vi "simple_RT_task.vi"(0 "stimulus length":u32=500 caption="Stimulus Length (ms)", 1 "monitor":u16 caption="Display", 5 "response window":u32=1000 caption="Response Window (ms)", 7 "ITI (ms)":u32=2000, 9 "file prefix":string caption="Output File Prefix", 11 "output folder":path caption="Output Folder", 12 "output channel":tag="Dev2/ao0" caption="Output Channel", 13 "randomization file":path) -> ()   [LabVIEW 2010]
uses:
  <vilib>/Utility/miscctls.llb/LVRectTypeDef.ctl
  <vilib>/Utility/miscctls.llb/LVPointTypeDef.ctl
  <vilib>/DAQmx/write.llb/DAQmx Write (Analog DBL 1Chan 1Samp).vi
  <vilib>/Utility/file.llb/Read From Spreadsheet File (DBL).vi
  <vilib>/DAQmx/create/channels.llb/DAQmx Create Channel (AO-Voltage-Basic).vi
  <vilib>/daqmx/miscellaneous.llb/DAQmx Fill In Error Info.vi
  <vilib>/Utility/inputDevices.llb/keyboardAcquire.vi
  <vilib>/Utility/inputDevices.llb/closeKeyboard.vi
panel:
  out "trial order":dbl[](array[numeric])
  out "old monitor":u16
  in  "Settings":enum32{"Page 1", "Page 2"}(tab)
  out "old panel bounds":T1
  out "output file ref":refnum<file>
  out "AO task id":refnum<k21>
  out "trial type":dbl
  out "response":T2(array[ring])
  out "response time":u32
  out "keyboard ID":refnum<k1>
  out "stimulus":string
  out "fixation":string
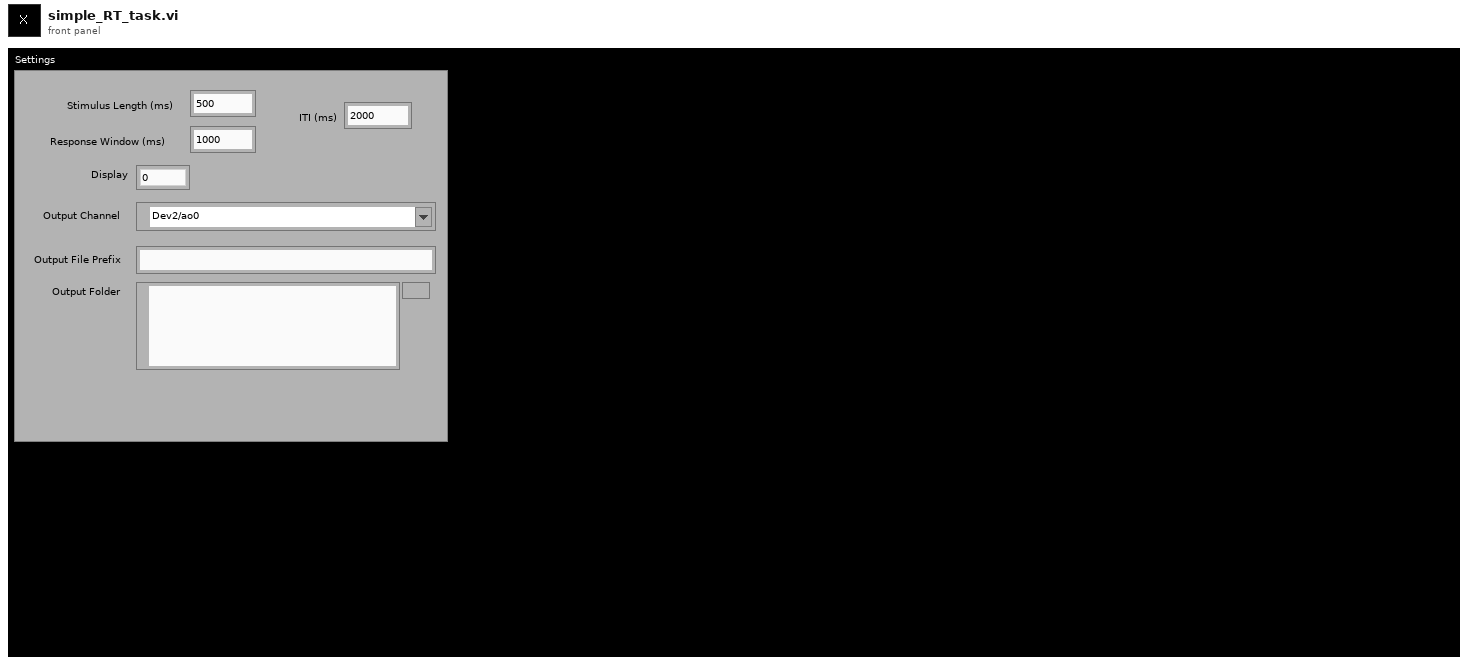
[diagram p1: front panel]
types:
  T1 = typedef "LVRectTypeDef.ctl" = cluster{"Left":i16, "Top":i16, "Right":i16, "Bottom":i16}
  T2 = enum16{"0", "1", "2", "3", "4", "5", "6", "7", "8", "9", "A", "B", "C", "D", "E", "F", "G", "H", "I", "J", "K", "L", "M", "N", "O", "P", "Q", "R", "S", "T", "U", "V", "W", "X", "Y", "Z", "F1", "F2", "F3", "F4", "F5", "F6", "F7", "F8", "F9", "F10", "F11", "F12", "F13", "F14", "F15", "ADD", "BACK", "BACKSLASH", "CAPITAL", "COMMA", "DECIMAL", "DELETE", "DIVIDE", "DOWN", "END", "EQUALS", "ESCAPE", "GRAVE (`)", "HOME", "INSERT", "LBRACKET", "LCONTROL", "LEFT", "L ALT", "LSHIFT", "LWIN", "MINUS", "MULTIPLY", "NEXT", "NUMLOCK", "NUMPAD_0", "NUMPAD_1", "NUMPAD_2", "NUMPAD_3", "NUMPAD_4", "NUMPAD_5", "NUMPAD_6", "NUMPAD_7", "NUMPAD_8", "NUMPAD_9", "PAUSE", "PERIOD", "PRIOR (PG UP)", "RBRACKET", "RCONTROL", "RETURN", "RIGHT", "R ALT", "RSHIFT", "RWIN", "SCROLL", "SEMICOLON", "SLASH", "SPACE", "SUBTRACT", "TAB", "UP", "ENTER (num pad)", "' (quote)"}[]
  T3 = enum16{"open", "replace", "create", "open or create", "replace or create", "replace or create with confirmation"}
  T4 = typedef "LVPointTypeDef.ctl" = cluster{"Horizontal":i16, "Vertical":i16}
  T5 = enum16{"0", "1", "2", "3", "4", "5", "6", "7", "8", "9", "A", "B", "C", "D", "E", "F", "G", "H", "I", "J", "K", "L", "M", "N", "O", "P", "Q", "R", "S", "T", "U", "V", "W", "X", "Y", "Z", "F1", "F2", "F3", "F4", "F5", "F6", "F7", "F8", "F9", "F10", "F11", "F12", "F13", "F14", "F15", "ADD", "BACK", "BACKSLASH", "CAPITAL", "COMMA", "DECIMAL", "DELETE", "DIVIDE", "DOWN", "END", "EQUALS", "ESCAPE", "GRAVE (`)", "HOME", "INSERT", "LBRACKET", "LCONTROL", "LEFT", "L ALT", "LSHIFT", "LWIN", "MINUS", "MULTIPLY", "NEXT", "NUMLOCK", "NUMPAD_0", "NUMPAD_1", "NUMPAD_2", "NUMPAD_3", "NUMPAD_4", "NUMPAD_5", "NUMPAD_6", "NUMPAD_7", "NUMPAD_8", "NUMPAD_9", "PAUSE", "PERIOD", "PRIOR (PG UP)", "RBRACKET", "RCONTROL", "RETURN", "RIGHT", "R ALT", "RSHIFT", "RWIN", "SCROLL", "SEMICOLON", "SLASH", "SPACE", "SUBTRACT", "TAB", "UP", "ENTER (num pad)", "' (quote)"}
  T6 = enum16{"big-endian, network order", "native, host order", "little-endian"}
  T7 = typedef "LVAllMonitorsDisplayTypeDef.ctl" = cluster{"Bounds":cluster{"Left":i16, "Top":i16, "Right":i16, "Bottom":i16}, "Depth":i16}[]
  T8 = cluster{"Bounds":cluster{"Left":i16, "Top":i16, "Right":i16, "Bottom":i16}, "Depth":i16}
  T9 = cluster{"Left":i16, "Top":i16, "Right":i16, "Bottom":i16}
  T10 = cluster{i32, "trial type":dbl, "response time":u32, "keyType 3":enum16{"0", "1", "2", "3", "4", "5", "6", "7", "8", "9", "A", "B", "C", "D", "E", "F", "G", "H", "I", "J", "K", "L", "M", "N", "O", "P", "Q", "R", "S", "T", "U", "V", "W", "X", "Y", "Z", "F1", "F2", "F3", "F4", "F5", "F6", "F7", "F8", "F9", "F10", "F11", "F12", "F13", "F14", "F15", "ADD", "BACK", "BACKSLASH", "CAPITAL", "COMMA", "DECIMAL", "DELETE", "DIVIDE", "DOWN", "END", "EQUALS", "ESCAPE", "GRAVE (`)", "HOME", "INSERT", "LBRACKET", "LCONTROL", "LEFT", "L ALT", "LSHIFT", "LWIN", "MINUS", "MULTIPLY", "NEXT", "NUMLOCK", "NUMPAD_0", "NUMPAD_1", "NUMPAD_2", "NUMPAD_3", "NUMPAD_4", "NUMPAD_5", "NUMPAD_6", "NUMPAD_7", "NUMPAD_8", "NUMPAD_9", "PAUSE", "PERIOD", "PRIOR (PG UP)", "RBRACKET", "RCONTROL", "RETURN", "RIGHT", "R ALT", "RSHIFT", "RWIN", "SCROLL", "SEMICOLON", "SLASH", "SPACE", "SUBTRACT", "TAB", "UP", "ENTER (num pad)", "' (quote)"}}
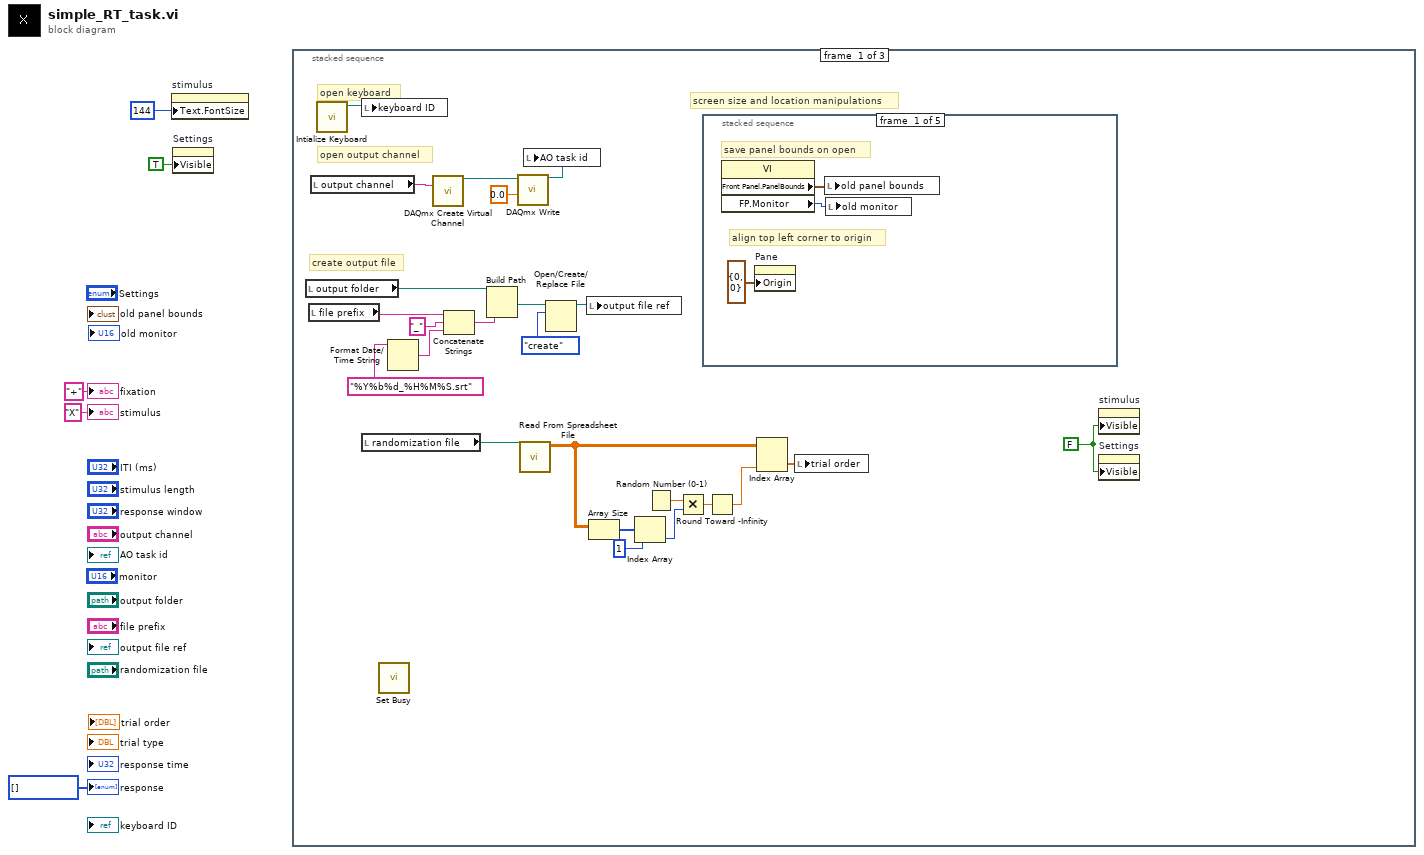
[diagram p0: block diagram]
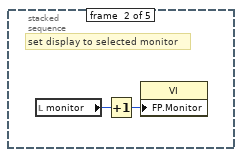
[diagram p2: hidden frame]
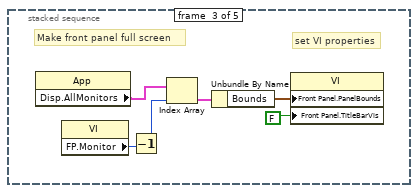
[diagram p3: hidden frame]
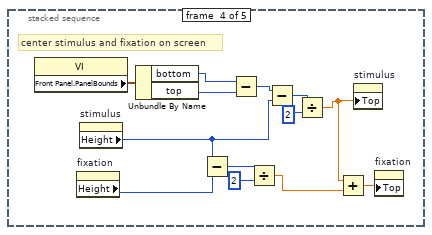
[diagram p4: hidden frame]
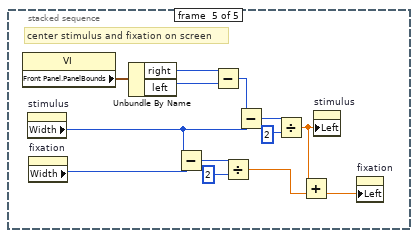
[diagram p5: hidden frame]
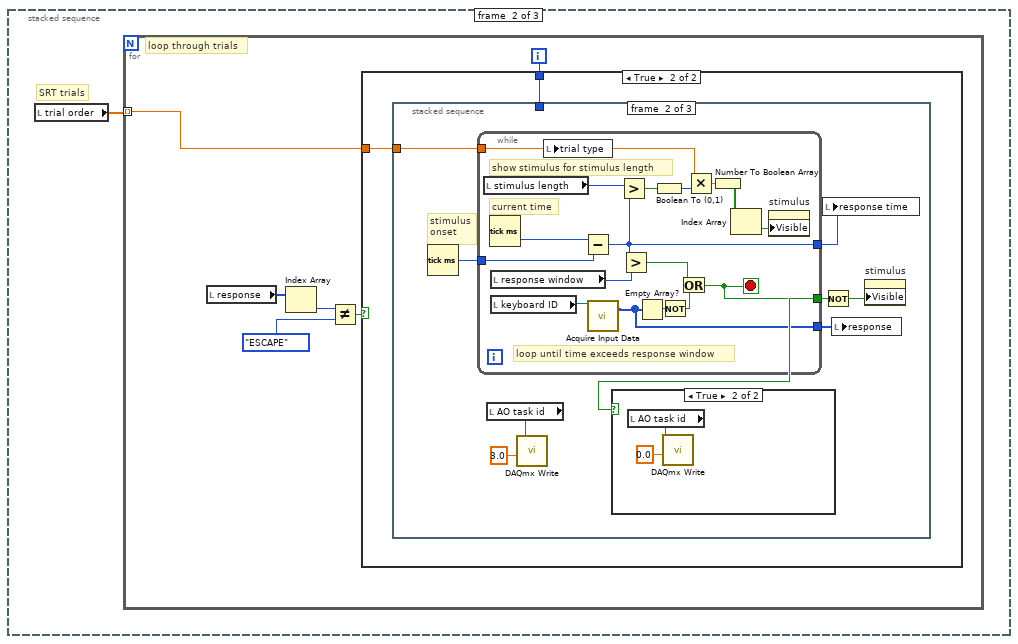
[diagram p6: hidden frame]
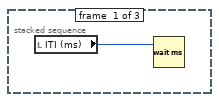
[diagram p8: hidden frame]
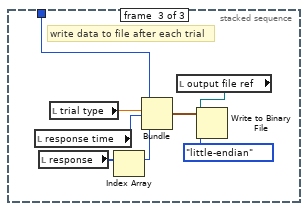
[diagram p10: hidden frame]
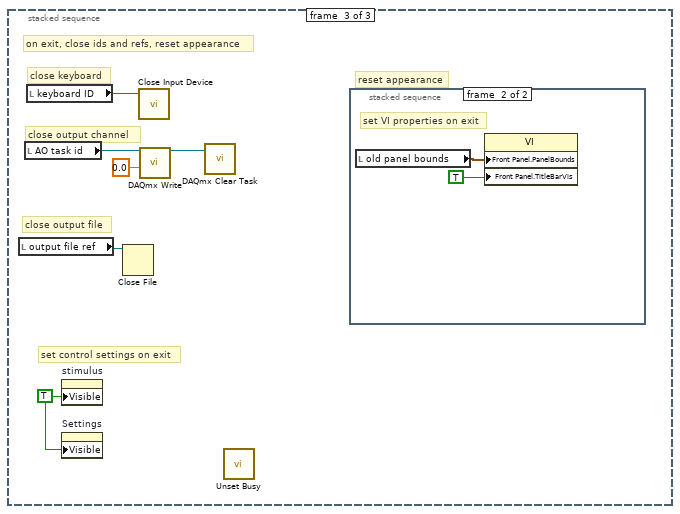
[diagram p11: hidden frame]
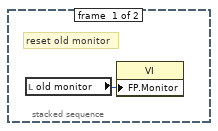
[diagram p12: hidden frame]
diagram:
  w1 = T2 [] items=["0", "1", "2", "3", "4", "5", "6", "7", "8", "9", "A", "B", "C", "D", "E", "F", "G", "H", "I", "J", "K", "L", "M", "N", "O", "P", "Q", "R", "S", "T", "U", "V", "W", "X", "Y", "Z", "F1", "F2", "F3", "F4", "F5", "F6", "F7", "F8", "F9", "F10", "F11", "F12", "F13", "F14", "F15", "ADD", "BACK", "BACKSLASH", "CAPITAL", "COMMA", "DECIMAL", "DELETE", "DIVIDE", "DOWN", "END", "EQUALS", "ESCAPE", "GRAVE (`)", "HOME", "INSERT", "LBRACKET", "LCONTROL", "LEFT", "L ALT", "LSHIFT", "LWIN", "MINUS", "MULTIPLY", "NEXT", "NUMLOCK", "NUMPAD_0", "NUMPAD_1", "NUMPAD_2", "NUMPAD_3", "NUMPAD_4", "NUMPAD_5", "NUMPAD_6", "NUMPAD_7", "NUMPAD_8", "NUMPAD_9", "PAUSE", "PERIOD", "PRIOR (PG UP)", "RBRACKET", "RCONTROL", "RETURN", "RIGHT", "R ALT", "RSHIFT", "RWIN", "SCROLL", "SEMICOLON", "SLASH", "SPACE", "SUBTRACT", "TAB", "UP", "ENTER (num pad)", "' (quote)"] ("response")
  n1 = property on="stimulus" class="Str"("Text.FontSize"=u32 144 ("Text.Font:Size")) -> ()  [unwired: 2 in, 2 out]
  n2 = property on="Settings" class="TabCtl (strict)"("Visible"=TRUE) -> ()  [unwired: 2 in, 2 out]
  n3 = stacked-sequence {
    frame #0 {
      w17 = FALSE ("Visible")
      # "screen size and location manipulations"
      # "create output file"
      # "open output channel"
      # "open keyboard"
      n4 = local read "output folder"() -> (w20:path)
      n5 = local read "file prefix"() -> (w21:string)
      n6 = local read "output channel"() -> (w27:tag)
      n7 = call <vilib>:"Intialize Keyboard.vi"() -> ("device ID"=w29:refnum<k1>)  [unwired: 10 in, 1 out]
      n8 = local write "keyboard ID"(w29) -> ()
      n9 = local read "randomization file"() -> (w12:path)
      n10 = call <vilib>:"Set Busy.vi"() -> ()  [unwired: 10 in, 2 out]
      n11 = Format Date/Time String(time format string (%c)="%Y%b%d_%H%M%S.srt") -> (date/time string=w7:string)  [unwired: 2 in]
      n12 = call-poly <vilib>:"DAQmx Create Virtual Channel.vi"("physical channels"=w27) -> ("task out"=w24:refnum<k21>)  [unwired: 13 in, 1 out]
      n13 = Concatenate Strings(w21, "_" ("string"), w7) -> (w19:string)
      n14 = Build Path(base path=w20, name or relative path=w19) -> (appended path=w18:path)
      n15 = call-poly <vilib>:"DAQmx Write.vi"("task/channels in"=w24, "data"=0.0) -> ("task out"=w23:refnum<k21>)  [unwired: 11 in, 2 out]
      n16 = call-poly <vilib>:"Read From Spreadsheet File.vi"("file path (dialog if empty)"=w12) -> ("all rows"=w11:dbl[][])  [unwired: 6 in, 4 out]
      n17 = local write "AO task id"(w23) -> ()
      n18 = Open/Create/Replace File(file path (use dialog)=w18, operation (0:open)=T3."create") -> (refnum out=w25:refnum<file>)  [unwired: 4 in, 2 out]
      n19 = local write "output file ref"(w25) -> ()
      n20 = Array Size(array=w11) -> (size(s)=w10:i32[])
      n21 = Index Array(array=w10, index=1) -> (element=w8:i32)
      n22 = Random Number (0-1)() -> (number: 0 to 1=w16:dbl)
      n23 = Multiply(x=w16, y=w8) -> (x*y=w15:dbl)
      n24 = stacked-sequence {
        frame #0 {
          # "align top left corner to origin"
          # "save panel bounds on open"
          n25 = property class="VI"() -> ("Front Panel.PanelBounds"=w32:T1, "FP.Monitor"=w30:u16)  [unwired: 2 in, 2 out]
          n26 = property on="Pane" class="Pane"("Origin"=T4 {"Horizontal"=0, "Vertical"=0}) -> ()  [unwired: 2 in, 2 out]
          n27 = local write "old panel bounds"(w32) -> ()
          n28 = local write "old monitor"(w30) -> ()
        }
        frame #1 {
          # "set display to selected monitor"
          n29 = local read "monitor"() -> (w34:u16)
          n30 = Increment(x=w34) -> (x+1=w33:u16)
          n31 = property class="VI"("FP.Monitor"=w33) -> ()  [unwired: 2 in, 2 out]
        }
        frame #2 {
          # "set VI properties"
          # "Make front panel full screen"
          n32 = property class="App"() -> ("Disp.AllMonitors"=w40:T7)  [unwired: 2 in, 2 out]
          n33 = property class="VI"() -> ("FP.Monitor"=w39:u16)  [unwired: 2 in, 2 out]
          n34 = Decrement(x=w39) -> (x-1=w38:u16)
          n35 = Index Array(array=w40, index=w38) -> (element=w37:T8)
          n36 = Unbundle By Name(w37) -> ("Bounds"=w36:T9)
          n37 = property class="VI"("Front Panel.PanelBounds"=w36, "Front Panel.TitleBarVis"=FALSE ("Front Panel Window:Title Bar Visible")) -> ()  [unwired: 2 in, 2 out]
        }
        frame #3 {
          # "center stimulus and fixation on screen"
          n38 = property class="VI"() -> ("Front Panel.PanelBounds"=w51:T1)  [unwired: 2 in, 2 out]
          n39 = property on="fixation" class="Str"() -> ("Height"=w44:u32)  [unwired: 2 in, 2 out]
          n40 = property on="stimulus" class="Str"() -> ("Height"=w45:u32)  [unwired: 2 in, 2 out]
          n41 = Unbundle By Name(w51) -> ("bottom"=w52:i16, "top"=w53:i16)
          n42 = Subtract(x=w45, y=w44) -> (x-y=w49:u32)
          n43 = Subtract(x=w52, y=w53) -> (x-y=w43:i16)
          n44 = Divide(x=w49, y=u32 2) -> (x/y=w46:dbl)
          n45 = Subtract(x=w43, y=w45) -> (x-y=w42:u32)
          n46 = Divide(x=w42, y=u32 2) -> (x/y=w41:dbl)
          n47 = Add(x=w41, y=w46) -> (x+y=w47:dbl)
          n48 = property on="stimulus" class="Str"("Top"=w41) -> ()  [unwired: 2 in, 2 out]
          n49 = property on="fixation" class="Str"("Top"=w47) -> ()  [unwired: 2 in, 2 out]
        }
        frame #4 {
          # "center stimulus and fixation on screen"
          n50 = property class="VI"() -> ("Front Panel.PanelBounds"=w66:T1)  [unwired: 2 in, 2 out]
          n51 = property on="stimulus" class="Str"() -> ("Width"=w57:u32)  [unwired: 2 in, 2 out]
          n52 = property on="fixation" class="Str"() -> ("Width"=w56:u32)  [unwired: 2 in, 2 out]
          n53 = Unbundle By Name(w66) -> ("right"=w64:i16, "left"=w65:i16)
          n54 = Subtract(x=w57, y=w56) -> (x-y=w60:u32)
          n55 = Subtract(x=w64, y=w65) -> (x-y=w63:i16)
          n56 = Divide(x=w60, y=u32 2) -> (x/y=w58:dbl)
          n57 = Subtract(x=w63, y=w57) -> (x-y=w61:u32)
          n58 = Divide(x=w61, y=u32 2) -> (x/y=w54:dbl)
          n59 = Add(x=w54, y=w58) -> (x+y=w55:dbl)
          n60 = property on="stimulus" class="Str"("Left"=w54) -> ()  [unwired: 2 in, 2 out]
          n61 = property on="fixation" class="Str"("Left"=w55) -> ()  [unwired: 2 in, 2 out]
        }
      }
      n62 = Round Toward -Infinity(1:w15) -> (0:w14:dbl)
      n63 = Index Array(array=w11, index (col)=w14) -> (element=w13:dbl[])  [unwired: 1 in]
      n64 = local write "trial order"(w13) -> ()
      n65 = property on="stimulus" class="Str"("Visible"=w17) -> ()  [unwired: 2 in, 2 out]
      n66 = property on="Settings" class="TabCtl (strict)"("Visible"=w17) -> ()  [unwired: 2 in, 2 out]
    }
    frame #1 {
      # "SRT trials"
      n67 = local read "trial order"() -> (w67:dbl[])
      n68 = for {
        tunnel: w67 -> [w72] mode=indexing
        i -> [w73]
        # "loop through trials"
        n69 = local read "response"() -> (w71:T2)
        n70 = Index Array(array=w71) -> (element=w70:T5)  [unwired: 1 in]
        n71 = Not Equal?(x=w70, y=T5."ESCAPE" ("element")) -> (x != y?=w68:bool)
        n72 = case shown="True" w68 {
          tunnel: w73 -> [_ w75]
          tunnel: w72 -> [_ w74]
          frame False {
          }
          frame True {
            n73 = stacked-sequence {
              tunnel: w75 -> [_ _ w105]
              tunnel: w74 -> [_ w77 _]
              frame #0 {
                n74 = local read "ITI (ms)"() -> (w76:u32)
                n75 = Wait (ms)(milliseconds to wait=w76) -> ()  [unwired: 1 out]
              }
              frame #1 {
                # "stimulus\nonset"
                n76 = Tick Count (ms)() -> (millisecond timer value=w82:u32)
                n77 = while {
                  tunnel: [w94] -> w84
                  tunnel: [w98] -> w83
                  tunnel: w82 -> [w97]
                  tunnel: [w93] -> w78
                  tunnel: w77 -> [w90]
                  stop <- w93 stop-if-true
                  # "show stimulus for stimulus length"
                  # "loop until time exceeds response window"
                  # "current time"
                  n78 = local read "stimulus length"() -> (w95:u32)
                  n79 = Tick Count (ms)() -> (millisecond timer value=w103:u32)
                  n80 = local read "response window"() -> (w96:u32)
                  n81 = local read "keyboard ID"() -> (w102:refnum<k1>)
                  n82 = local write "trial type"(w90) -> ()
                  n83 = Subtract(x=w103, y=w97) -> (x-y=w94:u32)
                  n84 = call-poly <vilib>:"Acquire Input Data.vi"("device ID"=w102) -> ("keys pressed"=w98:T2)  [unwired: 16 in, 2 out]
                  n85 = Greater?(x=w95, y=w94) -> (0:w92:bool)
                  n86 = Greater?(x=w94, y=w96) -> (0:w101:bool)
                  n87 = Empty Array?(array=w98) -> (empty?=w100:bool)
                  n88 = Boolean To (0,1)(Boolean=w92) -> (0, 1=w91:i16)
                  n89 = Not(x=w100) -> (.not. x?=w99:bool)
                  n90 = Or(x=w101, y=w99) -> (x .or. y?=w93:bool)
                  n91 = Multiply(x=w90, y=w91) -> (x*y=w89:dbl)
                  n92 = Number To Boolean Array(number=w89) -> (Boolean array=w88:bool[])
                  n93 = Index Array(array=w88) -> (element=w87:bool)  [unwired: 1 in]
                  n94 = property on="stimulus" class="Str"("Visible"=w87) -> ()  [unwired: 2 in, 2 out]
                }
                n95 = local read "AO task id"() -> (w80:refnum<k21>)
                n96 = call-poly <vilib>:"DAQmx Write.vi"("task/channels in"=w80, "data"=3.0) -> ()  [unwired: 11 in, 3 out]
                n97 = case shown="True" w78 {
                  frame False {
                  }
                  frame True {
                    n98 = local read "AO task id"() -> (w85:refnum<k21>)
                    n99 = call-poly <vilib>:"DAQmx Write.vi"("task/channels in"=w85, "data"=0.0) -> ()  [unwired: 11 in, 3 out]
                  }
                }
                n100 = local write "response time"(w84) -> ()
                n101 = Not(x=w78) -> (.not. x?=w81:bool)
                n102 = local write "response"(w83) -> ()
                n103 = property on="stimulus" class="Str"("Visible"=w81) -> ()  [unwired: 2 in, 2 out]
              }
              frame #2 {
                # "write data to file after each trial"
                n104 = local read "response time"() -> (w111:u32)
                n105 = local read "response"() -> (w110:T2)
                n106 = local read "trial type"() -> (w104:dbl)
                n107 = Index Array(array=w110) -> (element=w109:T5)  [unwired: 1 in]
                n108 = Bundle(w105, "trial type"=w104, "response time"=w111, "keyType 3"=w109) -> (w107:T10)  [unwired: 1 in]
                n109 = local read "output file ref"() -> (w106:refnum<file>)
                n110 = Write to Binary File(file (use dialog)=w106, data=w107, 9:T6."little-endian" ("byte order (0:big-endian, network order)")) -> ()  [unwired: 3 in, 3 out]
              }
            }
          }
        }
      }
    }
    frame #2 {
      w112 = TRUE ("Visible")
      # "reset appearance"
      # "on exit, close ids and refs, reset appearance"
      # "set control settings on exit"
      # "close output file"
      # "close output channel"
      # "close keyboard"
      n111 = local read "output file ref"() -> (w113:refnum<file>)
      n112 = local read "AO task id"() -> (w116:refnum<k21>)
      n113 = local read "keyboard ID"() -> (w117:refnum<k1>)
      n114 = property on="stimulus" class="Str"("Visible"=w112) -> ()  [unwired: 2 in, 2 out]
      n115 = property on="Settings" class="TabCtl (strict)"("Visible"=w112) -> ()  [unwired: 2 in, 2 out]
      n116 = Close File(refnum=w113) -> ()  [unwired: 1 in, 2 out]
      n117 = call-poly <vilib>:"Close Input Device.vi"("device ID"=w117) -> ()  [unwired: 9 in, 1 out]
      n118 = call-poly <vilib>:"DAQmx Write.vi"("task/channels in"=w116, "data"=0.0) -> ("task out"=w115:refnum<k21>)  [unwired: 11 in, 2 out]
      n119 = call <vilib>:"DAQmx Clear Task.vi"("task in"=w115) -> ()  [unwired: 14 in, 1 out]
      n120 = call <vilib>:"Unset Busy.vi"() -> ()  [unwired: 11 in, 1 out]
      n121 = stacked-sequence {
        frame #0 {
          # "reset old monitor"
          n122 = local read "old monitor"() -> (w118:u16)
          n123 = property class="VI"("FP.Monitor"=w118) -> ()  [unwired: 2 in, 2 out]
        }
        frame #1 {
          # "set VI properties on exit"
          n124 = local read "old panel bounds"() -> (w119:T1)
          n125 = property class="VI"("Front Panel.PanelBounds"=w119, "Front Panel.TitleBarVis"=TRUE ("Front Panel Window:Title Bar Visible")) -> ()  [unwired: 2 in, 2 out]
        }
      }
    }
  }
  "stimulus" <- "X" ("stimulus")
  "response" <- w1
  "fixation" <- "+" ("fixation")
